vi "Get all controls from list of controls.vi"(8 "error in":errorcluster, 9 "Exclude tabs?":bool, 10 "VI Panel":refnum<vi>) -> (0 "error out":errorcluster, 2 "All Controls (except/incl tabs) []":refnum<vi>[](array[refnum]), 3 "VI Panel refout":refnum<vi>)   [LabVIEW 2013]
doc: "This .vi recursively finds all controls including those within tabs (and nested tabs) from the input VI panel. The tab controls can be selectively added or excluded from output."
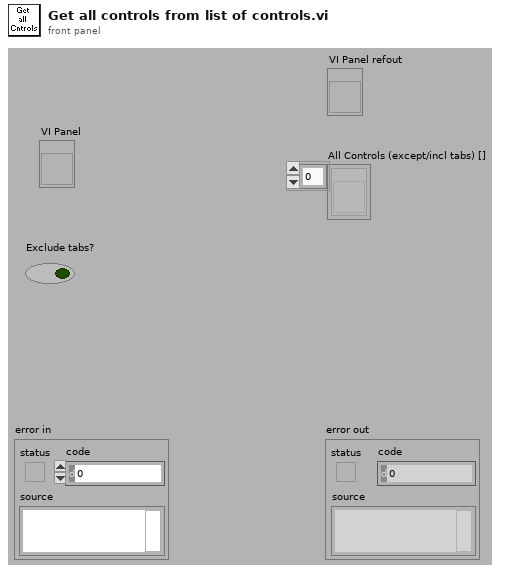
[diagram p1: front panel]
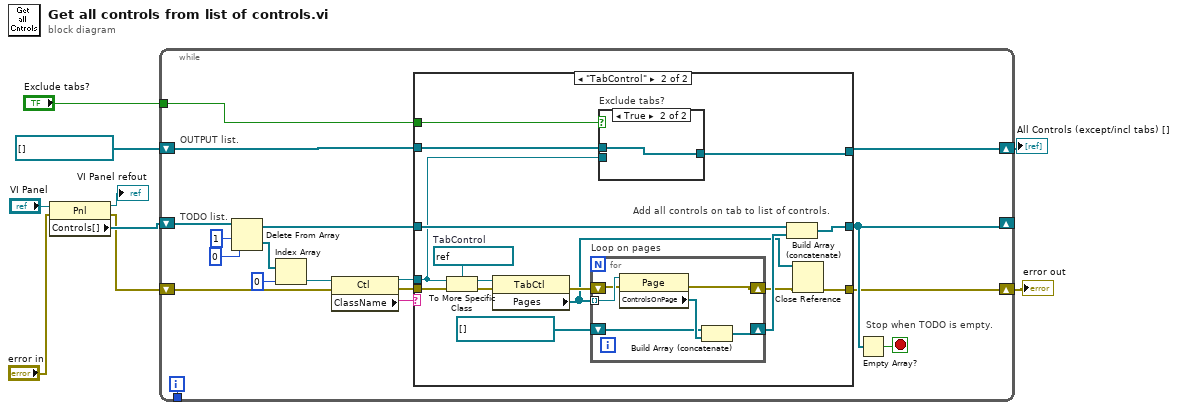
[diagram p0: block diagram]
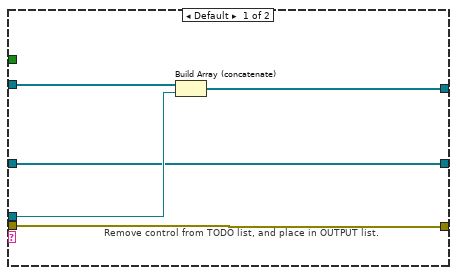
[diagram p2: hidden frame]
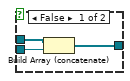
[diagram p3: hidden frame]
diagram:
  n1 = property class="Pnl"(reference="VI Panel", error in="error in") -> (reference out=→"VI Panel refout":refnum<vi>, error out=w3:errorcluster, "Controls[]"=w4:refnum<vi>[])
  n2 = while {
    shift-right: [w22] -> _
    shift-left: w4 -> [w16]
    shift-right: [w25] -> w8
    shift-left: refnum<vi>[] [] -> [w24]
    tunnel: "Exclude tabs?" -> [w12]
    tunnel: [w10] -> _
    shift-right: [w19] -> w7
    shift-left: w3 -> [w11]
    i -> [w10]
    stop <- w23 stop-if-true
    # "OUTPUT list."
    # "TODO list."
    # "Stop when TODO is empty."
    n3 = Delete From Array "Delete From Array"(array=w16, length=1, index=0) -> (deleted portion=w15:refnum<vi>[], array with subset deleted=w13:refnum<vi>[])
    n4 = Index Array(array=w15, index=0) -> (element=w21:refnum<vi>)
    n5 = property class="Ctl"(reference=w21, error in=w11) -> (reference out=w26:refnum<vi>, error out=w20:errorcluster, "ClassName"=w27:string)
    n6 = case shown="\"TabControl\"" w27 {
      tunnel: w26 -> [w29 w36]
      tunnel: w13 -> [w28 w44]
      tunnel: [w31 w37] -> w25
      tunnel: w24 -> [w32 w38]
      tunnel: [w28 w45] -> w22
      tunnel: w20 -> [w30 w41]
      tunnel: [w30 w34] -> w19
      tunnel: w12 -> [_ w39]
      frame Default {
        # "Remove control from TODO list, and place in OUTPUT list."
        n7 = Build Array (concatenate)(w32, w29) -> (w31:refnum<vi>[])
      }
      frame "TabControl" {
        w48 = refnum<vi> refnum  # TabControl
        # "Add all controls on tab to list of controls."
        n8 = To More Specific Class(target class=w48, reference=w36, error in=w41) -> (specific class reference=w46:refnum<vi>, error out=w47:errorcluster)
        n9 = property class="TabCtl"(reference=w46, error in=w47) -> (error out=w40:errorcluster, "Pages"=w33:refnum<vi>[])  [unwired: 1 out]
        n10 = for "Loop on pages" {
          tunnel: w33 -> [w58] mode=indexing
          shift-right: [w55] -> w42
          shift-left: refnum<vi>[] [] -> [w56]
          shift-right: [w53] -> w35
          shift-left: w40 -> [w54]
          n11 = property class="Page"(reference=w58, error in=w54) -> (error out=w53:errorcluster, "ControlsOnPage"=w57:refnum<vi>[])  [unwired: 1 out]
          n12 = Build Array (concatenate)(w56, w57) -> (w55:refnum<vi>[])
        }
        n13 = case "Exclude tabs?" shown="True" w39 {
          tunnel: w36 -> [w51 _]
          tunnel: w38 -> [w50 w52]
          tunnel: [w49 w52] -> w37
          frame False {
            n14 = Build Array (concatenate)(w50, w51) -> (w49:refnum<vi>[])
          }
          frame True {
          }
        }
        n15 = Build Array (concatenate)(w44, w42) -> (w45:refnum<vi>[])
        n16 = Close Reference(reference=w33, error in (no error)=w35) -> (error out=w34:errorcluster)
      }
    }
    n17 = Empty Array?(array=w22) -> (empty?=w23:bool)
  }
  "error out" <- w7
  "All Controls (except/incl tabs) []" <- w8
